vi "Main.vi"() -> ()   [LabVIEW 2018]
uses:
  Main_SubVI/Progress.vi
  <vilib>/Utility/file.llb/Write Delimited Spreadsheet (DBL).vi
panel:
  out "error out":errorcluster
  out "Progress Output":string
  out "Progress":u8(slide) scale=0.0..100.0
  out "Arduino Conn":bool
  in  "Arduino Connection":T1={"Baud rate (115200)"=115200, "VISA resource name"="", "Disconnect"=FALSE} {"Baud rate (115200)" min=38400 max=500000 step=1}
  out "Monitor":T2 {"Elapsed time [s]" format="%#_1g"}
  in  "Tab Plot":enum32{"Plot Measure", "Calibration Settings"}(tab)
  out "Measure VS Distance Reference":cluster{dbl[], dbl[]}(graph)
  out "Distance Sample":T3(graph)
  in  "Calibration":bool
  in  "Auto Validation":bool
  in  "Tare":bool
  in  "Reset Calibration":bool
  out "Calibration Curve":cluster{"Best Linear Fit":dbl[], dbl[]}[](graph)
  out "Calibration parameters":T4
  in  "Save Calibration":bool
  out "Measure":T5 {"Arduino distance [mm]" format="%#_5g"}
  in  "Tab Control":enum32{"Manual", " Programmable"}(tab)
  in  "Stop 2":bool
  out "Motor Ready":bool
  out "Communication\nAcknowledged":bool
  in  "Direction":bool
  in  "Motor relative position [mm]":dbl(knob) min=0.0 max=199.89999389648438 step=0.1 scale=0.0..100.0
  in  "Start Communication":bool
  in  "Samples per position":i32=1 min=1 step=1
  in  "Import":path
  in  "Start Auto Communication":bool
  in  "Stop":bool
  out "VISA resource name out":refnum<visa-resource-name>
  # "%"
  # "Up"
  # "Down"
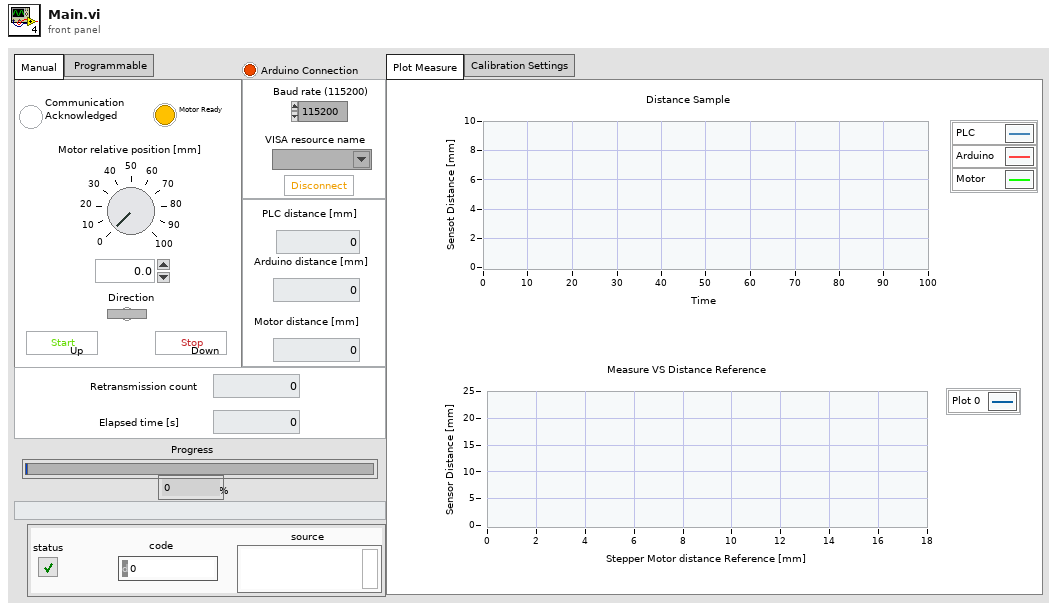
[diagram p1: front panel]
types:
  T1 = cluster{"Baud rate (115200)":u32, "VISA resource name":refnum<visa-resource-name>, "Disconnect":bool}
  T2 = cluster{"Elapsed time [s]":dbl, "Retransmission count":dbl}
  T3 = cluster{"PLC Sensor":dbl, "Arduino Sensor":dbl, "Position Reference":dbl}
  T4 = cluster{"Gain":dbl, "Offset":dbl, "ERMS":dbl, "STD":dbl, "Samples ":dbl}
  T5 = cluster{"PLC distance [mm] ":dbl, "Arduino distance [mm]":dbl, "Motor distance [mm]":dbl}
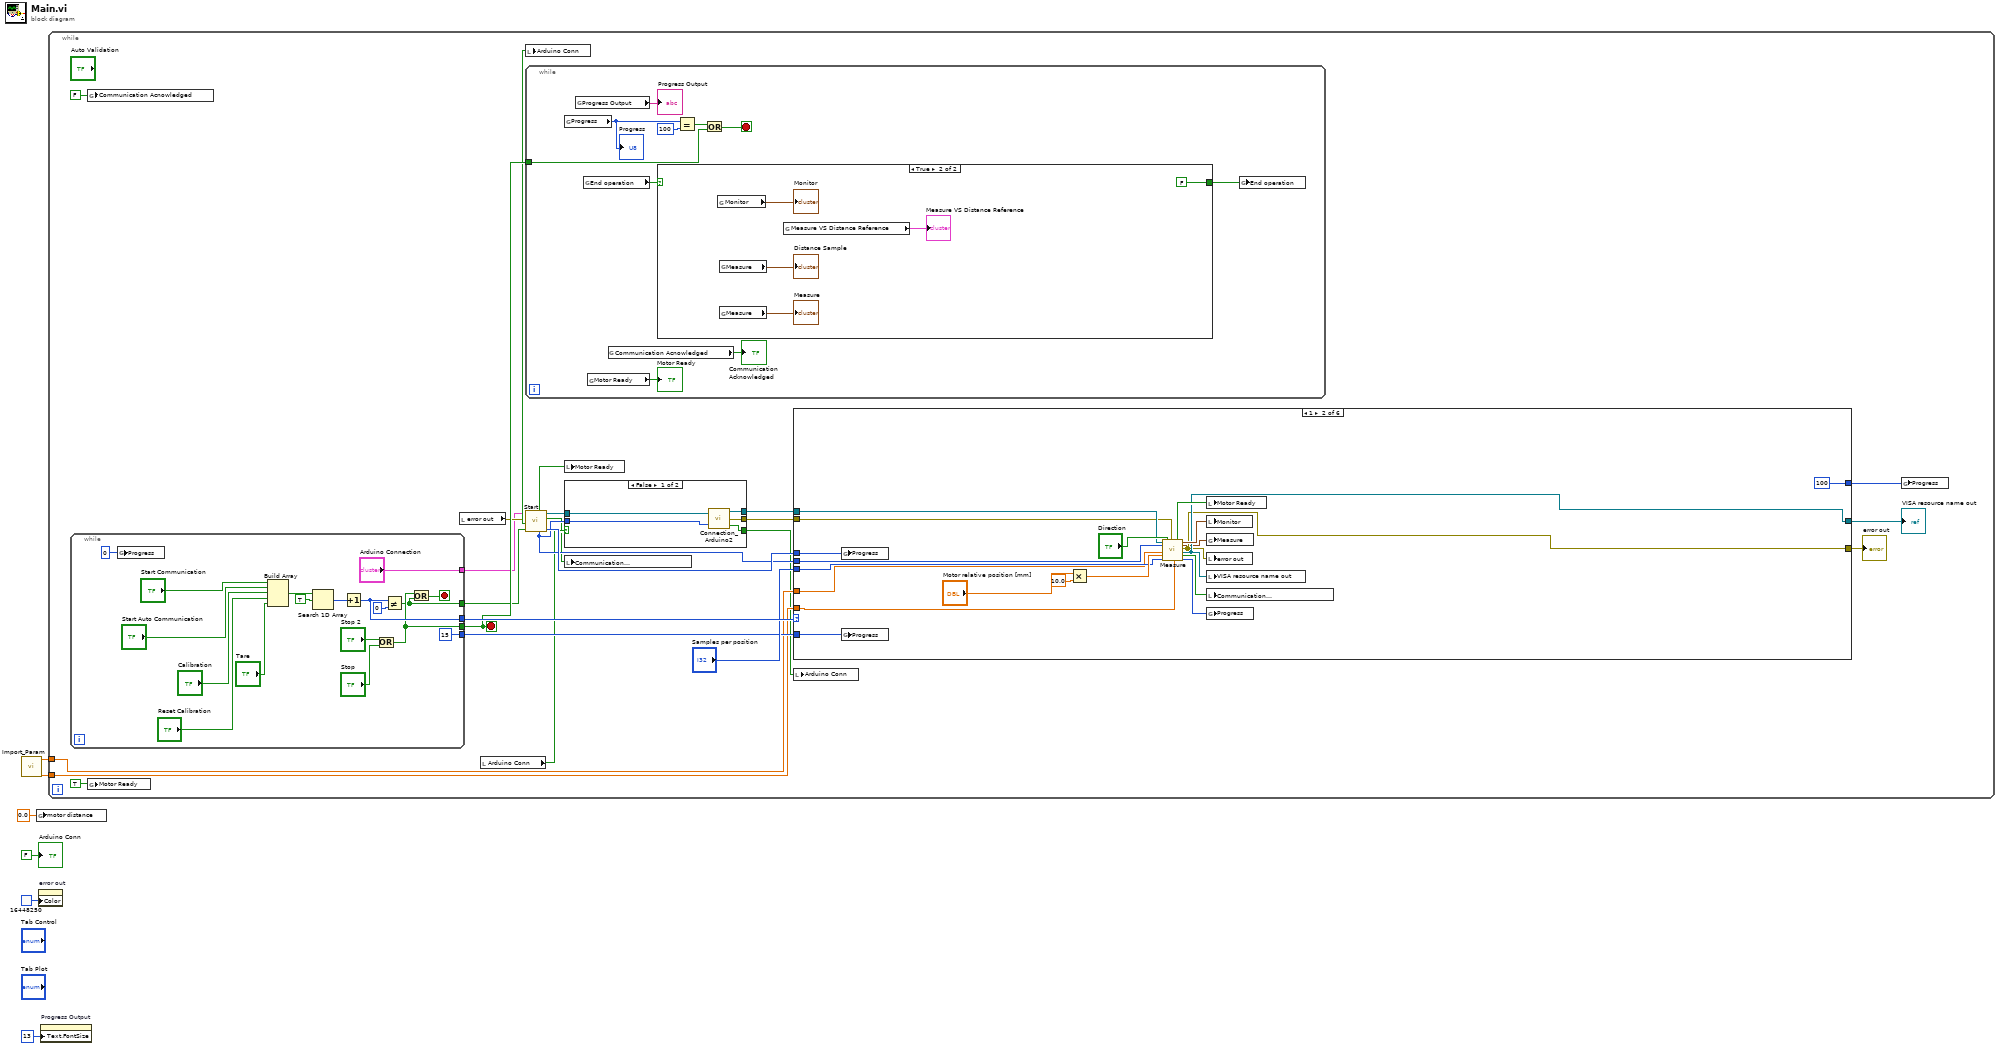
[diagram p0: block diagram]
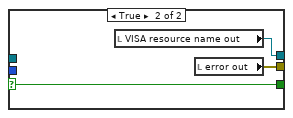
[diagram p2: hidden frame]
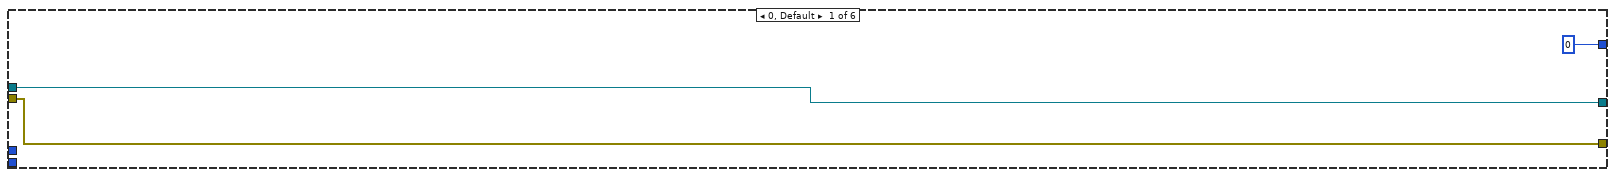
[diagram p3: hidden frame]
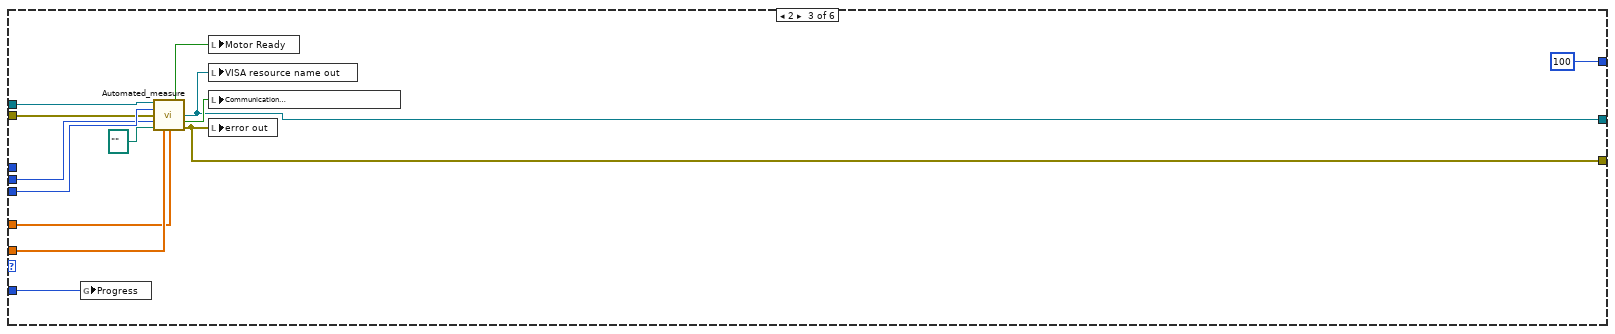
[diagram p4: hidden frame]
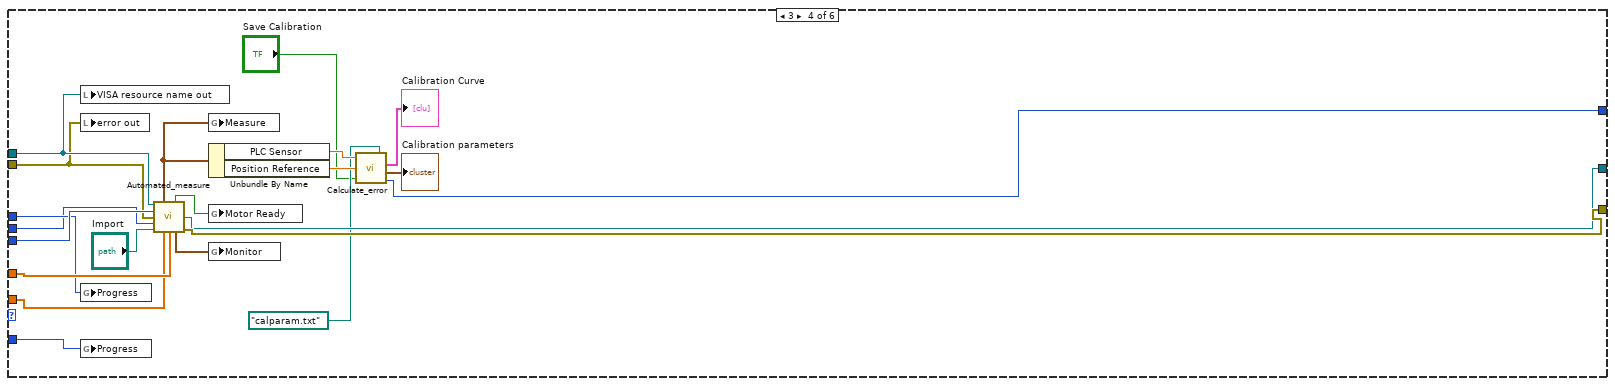
[diagram p5: hidden frame]
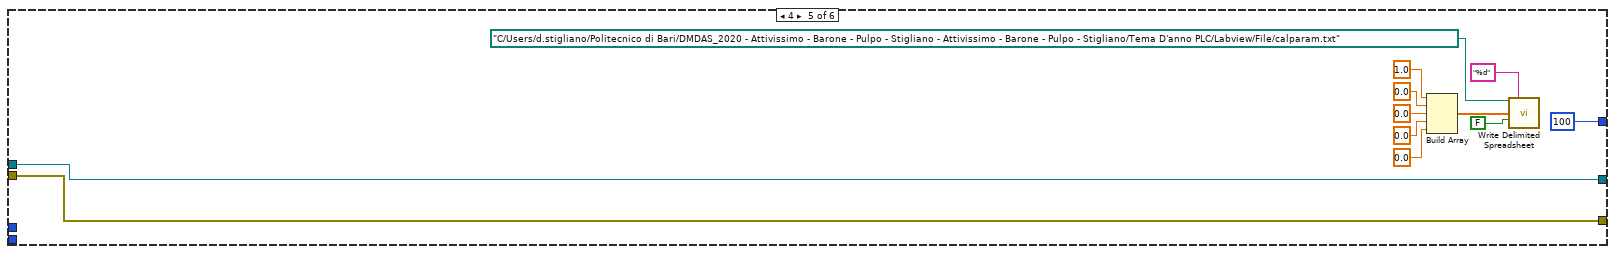
[diagram p6: hidden frame]
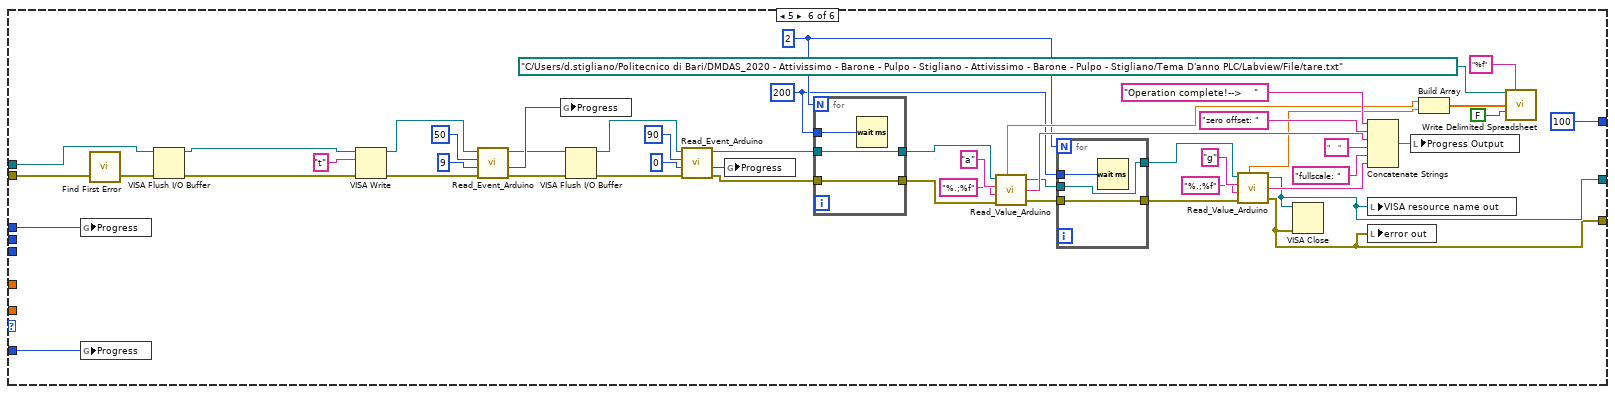
[diagram p7: hidden frame]
diagram:
  n1 = call "Import_Param.vi"() -> ("Calparam"=w5:sgl[], "Initial Tare"=w6:sgl[])  [unwired: 2 out]
  n2 = global write "Progress.vi" "motor distance"(0.0 ("motor distance")) -> ()
  n3 = property on="error out" class="Clust (strict)"("Color"=u32 16448250) -> ()  [unwired: 2 in, 2 out]
  n4 = property on="Progress Output" class="Str"("Text.FontSize"=u32 13 ("Text.Font:Size")) -> ()  [unwired: 2 in, 2 out]
  n5 = while {
    tunnel: w6 -> [w25]
    tunnel: w5 -> [w24]
    stop <- w28 stop-if-true
    n6 = while {
      tunnel: [u8 15 ("Slide")] -> w27
      tunnel: [w48] -> w30
      tunnel: [w43] -> w28
      tunnel: ["Arduino Connection"] -> w8
      tunnel: [w39] -> w7
      stop <- w40 stop-if-true
      n7 = global write "Progress.vi" "Progress"(u8 0 ("Slide")) -> ()
      n8 = Build Array("Start Communication", "Start Auto Communication", "Calibration", "Reset Calibration", "Tare") -> (w56:bool[])
      n9 = Search 1D Array(1D array=w56, element=TRUE) -> (index of element=w54:i32)  [unwired: 1 in]
      n10 = Increment(x=w54) -> (x+1=w48:i32)
      n11 = Or(x="Stop 2", y="Stop") -> (x .or. y?=w43:bool)
      n12 = Not Equal?(x=w48, y=0) -> (x != y?=w39:bool)
      n13 = Or(x=w43, y=w39) -> (x .or. y?=w40:bool)
    }
    n14 = global write "Progress.vi" "Communication Acnowledged"(FALSE ("Communication")) -> ()
    n15 = global write "Progress.vi" "Motor Ready"(TRUE ("Communication")) -> ()
    n16 = local read "error out"() -> (w9:errorcluster)
    n17 = local read "Arduino Conn"() -> (w15:bool)
    n18 = while {
      tunnel: w28 -> [w187]
      stop <- w189 stop-if-true
      n19 = global read "Progress.vi" "Progress"() -> (w191:u8)
      "Progress" <- w191
      n20 = global read "Progress.vi" "Progress Output"() -> (→"Progress Output":string)
      n21 = global read "Progress.vi" "End operation"() -> (w183:bool)
      n22 = global read "Progress.vi" "Motor Ready"() -> (→"Motor Ready":bool)
      n23 = global read "Progress.vi" "Communication Acnowledged"() -> (→"Communication\nAcknowledged":bool)
      n24 = case shown="True" w183 {
        selector: w183 -> [w192 _]
        tunnel: [w192 FALSE ("End operation")] -> w182
        frame False {
        }
        frame True {
          n25 = global read "Progress.vi" "Monitor"() -> (→"Monitor":T2)
          n26 = global read "Progress.vi" "Measure"() -> (→"Distance Sample":T5)
          n27 = global read "Progress.vi" "Measure"() -> (→"Measure":T5)
          n28 = global read "Progress.vi" "Measure VS Distance Reference"() -> (→"Measure VS Distance Reference":cluster{dbl[], dbl[]})
        }
      }
      n29 = Equal?(x=w191, y=u8 100) -> (x = y?=w188:bool)
      n30 = Or(x=w188, y=w187) -> (x .or. y?=w189:bool)
      n31 = global write "Progress.vi" "End operation"(w182) -> ()
    }
    n32 = call "Start.vi"("Arduino Connection"=w8, "error in (no error)"=w9, "Start Communication"=w7) -> ("Arduino Conn"=w17:bool, "Motor Ready"=w22:bool, "Baud rate (115200)"=w19:u32, "VISA resource name"=w16:refnum<visa-resource-name>, "Communication"=w14:bool, "Slide"=w23:u8)  [unwired: 1 out]
    n33 = local write "Arduino Conn"(w17) -> ()
    n34 = local write "Motor Ready"(w22) -> ()
    n35 = case shown="False" w15 {
      selector: w15 -> [_ w36]
      tunnel: w19 -> [w35 _]
      tunnel: [w34 w38] -> w20
      tunnel: [w33 w37] -> w21
      tunnel: [w32 w36] -> w18
      tunnel: w16 -> [w31 _]
      frame False {
        n36 = call "Connection_Arduino2.vi"("VISA resource name"=w31, "baud rate (9600)"=w35) -> ("VISA resource name out"=w34:refnum<visa-resource-name>, "error out"=w33:errorcluster, "Arduino Conn"=w32:bool)
      }
      frame True {
        n37 = local read "VISA resource name out"() -> (w38:refnum<visa-resource-name>)
        n38 = local read "error out"() -> (w37:errorcluster)
      }
    }
    n39 = local write "Communication\nAcknowledged"(w14) -> ()
    n40 = case shown="1" w30 {
      tunnel: "Samples per position" -> [_ w74 w90 w112 _ _]
      tunnel: w27 -> [_ w73 w89 w111 _ w169]
      tunnel: [u8 0 ("Progress") u8 100 ("Progress") u8 100 ("Progress") w93 u8 100 ("Progress") u8 100 ("Progress")] -> w26
      tunnel: w25 -> [_ w72 w86 w110 _ _]
      tunnel: w24 -> [_ w71 w87 w109 _ _]
      tunnel: w23 -> [_ w70 _ w108 _ w130]
      tunnel: w20 -> [w58 w69 w81 w106 w115 w129]
      tunnel: w21 -> [w57 w67 w83 w105 w114 w128]
      tunnel: w19 -> [_ w68 w84 w107 _ _]
      tunnel: [w57 w63 w82 w103 w114 w126] -> w13
      tunnel: [w58 w64 w80 w102 w115 w127] -> w12
      frame 0, Default {
      }
      frame 1 {
        n41 = global write "Progress.vi" "Progress"(w70) -> ()
        n42 = global write "Progress.vi" "Progress"(w73) -> ()
        n43 = Multiply(x="Motor relative position [mm]", y=10.0) -> (x*y=w79:dbl)
        n44 = call "Measure.vi"("VISA resource name"=w69, "Baud rate (115200)"=w68, "Initial Tare"=w72, "Motor relative position"=w79, "Samples per position"=w74, "Direction"="Direction", "error in"=w67, "Cal Param"=w71) -> ("Motor Ready"=w66:bool, "Monitor"=w77:T2, "Measure"=w62:T5, "error out"=w63:errorcluster, "VISA resource name out"=w64:refnum<visa-resource-name>, "Communication\nAcknowledged"=w65:bool, "Progress"=w61:u8)  [unwired: 5 in]
        n45 = local write "Motor Ready"(w66) -> ()
        n46 = local write "Monitor"(w77) -> ()
        n47 = global write "Progress.vi" "Measure"(w62) -> ()
        n48 = local write "error out"(w63) -> ()
        n49 = local write "VISA resource name out"(w64) -> ()
        n50 = local write "Communication\nAcknowledged"(w65) -> ()
        n51 = global write "Progress.vi" "Progress"(w61) -> ()
      }
      frame 2 {
        n52 = global write "Progress.vi" "Progress"(w89) -> ()
        n53 = call "Automated_measure.vi"("VISA resource name"=w81, "Samples per position"=w90, "error in"=w83, "Baud rate (115200)"=w84, "Import"=path "", "Cal Param"=w87, "Initial Tare"=w86) -> ("Motor Ready"=w92:bool, "VISA resource name out"=w80:refnum<visa-resource-name>, "Communication OK"=w85:bool, "error out"=w82:errorcluster)  [unwired: 3 in, 2 out]
        n54 = local write "Motor Ready"(w92) -> ()
        n55 = local write "VISA resource name out"(w80) -> ()
        n56 = local write "Communication\nAcknowledged"(w85) -> ()
        n57 = local write "error out"(w82) -> ()
      }
      frame 3 {
        n58 = local write "VISA resource name out"(w106) -> ()
        n59 = local write "error out"(w105) -> ()
        n60 = global write "Progress.vi" "Progress"(w108) -> ()
        n61 = global write "Progress.vi" "Progress"(w111) -> ()
        n62 = call "Automated_measure.vi"("VISA resource name"=w106, "Samples per position"=w112, "error in"=w105, "Baud rate (115200)"=w107, "Import"="Import", "Cal Param"=w109, "Initial Tare"=w110) -> ("Measure"=w94:T3, "Motor Ready"=w104:bool, "VISA resource name out"=w102:refnum<visa-resource-name>, "Monitor"=w101:T2, "error out"=w103:errorcluster)  [unwired: 3 in, 1 out]
        n63 = global write "Progress.vi" "Measure"(w94) -> ()
        n64 = Unbundle By Name(w94) -> ("PLC Sensor"=w97:dbl, "Position Reference"=w98:dbl)
        n65 = global write "Progress.vi" "Motor Ready"(w104) -> ()
        n66 = global write "Progress.vi" "Monitor"(w101) -> ()
        n67 = call "Calculate_error.vi"("x 2"=w97, "x 1"=w98, "Button"="Save Calibration", "file path (dialog if empty)"=path "calparam.txt") -> ("Calibration Curve"=→"Calibration Curve":cluster{"Best Linear Fit":dbl[], dbl[]}[], "Calibration parameters"=→"Calibration parameters":T4, "Slide"=w93:u8)
      }
      frame 4 {
        n68 = Build Array(1.0 ("element"), 0.0 ("element"), 0.0 ("element"), 0.0 ("element"), 0.0 ("element")) -> (w116:dbl[])
        n69 = call-poly <vilib>:"Write Delimited Spreadsheet.vi"("file path (dialog if empty)"=path "C:/Users/d.stigliano/Politecnico di Bari/DMDAS_2020 - Attivissimo - Barone - Pulpo - Stigliano - Attivissimo - Barone - Pulpo - Stigliano/Tema D'anno PLC/Labview/File/calparam.txt", "format (%.3f)"="%d", "1D data"=w116, "append to file? (new file:F)"=FALSE) -> ()  [unwired: 10 in, 2 out]
      }
      frame 5 {
        w133 = u32 200 ("milliseconds to wait")
        w135 = 2
        n70 = global write "Progress.vi" "Progress"(w130) -> ()
        n71 = global write "Progress.vi" "Progress"(w169) -> ()
        n72 = call <vilib>:"Find First Error.vi"("error in (no error)"=w128) -> ("error out"=w172:errorcluster)  [unwired: 3 in, 1 out]
        n73 = VISA Flush I/O Buffer(VISA resource name=w129, error in (no error)=w172) -> (VISA resource name out=w168:refnum<visa-resource-name>, error out=w171:errorcluster)  [unwired: 1 in]
        n74 = VISA Write(VISA resource name=w168, write buffer="t", error in (no error)=w171) -> (VISA resource name out=w165:refnum<visa-resource-name>, error out=w164:errorcluster)  [unwired: 1 out]
        n75 = call "Read_Event_Arduino.vi"("error in"=w164, "condition"=9, "Progress in"=u8 50 ("Progress"), "VISA resource name in"=w165) -> ("error out"=w155:errorcluster, "Progress"=w163:u8, "VISA resource name out"=w157:refnum<visa-resource-name>)  [unwired: 4 in, 1 out]
        n76 = global write "Progress.vi" "Progress"(w163) -> ()
        n77 = VISA Flush I/O Buffer(VISA resource name=w157, error in (no error)=w155) -> (VISA resource name out=w156:refnum<visa-resource-name>, error out=w154:errorcluster)  [unwired: 1 in]
        n78 = call "Read_Event_Arduino.vi"("error in"=w154, "condition"=0, "Progress in"=u8 90, "VISA resource name in"=w156) -> ("error out"=w143:errorcluster, "Progress"=w162:u8, "VISA resource name out"=w146:refnum<visa-resource-name>)  [unwired: 4 in, 1 out]
        n79 = global write "Progress.vi" "Progress"(w162) -> ()
        n80 = for {
          N: w135 -> [_]
          tunnel: w146 -> [w181]
          tunnel: [w181] -> w145
          tunnel: [w180] -> w144
          tunnel: w143 -> [w180]
          tunnel: w133 -> [w179]
          n81 = Wait (ms)(milliseconds to wait=w179) -> ()  [unwired: 1 out]
        }
        n82 = call "Read_Value_Arduino.vi"("VISA resource name"=w145, "write buffer"="a", "format string (%.;%f)"="%.;%f" ("format string (%d)"), "error in (no error)"=w144) -> ("output"=w147:dbl, "VISA resource name out"=w142:refnum<visa-resource-name>, "concatenated string"=w149:string, "error out"=w141:errorcluster)
        n83 = for {
          N: w135 -> [_]
          tunnel: w142 -> [w177]
          tunnel: [w178] -> w140
          tunnel: w141 -> [w178]
          tunnel: [w177] -> w139
          tunnel: w133 -> [w176]
          n84 = Wait (ms)(milliseconds to wait=w176) -> ()  [unwired: 1 out]
        }
        n85 = call "Read_Value_Arduino.vi"("VISA resource name"=w139, "write buffer"="g", "format string (%.;%f)"="%.;%f" ("format string (%d)"), "error in (no error)"=w140) -> ("output"=w148:dbl, "VISA resource name out"=w127:refnum<visa-resource-name>, "concatenated string"=w138:string, "error out"=w126:errorcluster)
        n86 = VISA Close(VISA resource name=w127, error in (no error)=w126) -> ()  [unwired: 1 out]
        n87 = Concatenate Strings("Operation complete!-->    " ("string"), "zero offset: " ("string"), w149, "    " ("string"), "fullscale: " ("string"), w138) -> (w132:string)
        n88 = local write "VISA resource name out"(w127) -> ()
        n89 = local write "error out"(w126) -> ()
        n90 = local write "Progress Output"(w132) -> ()
        n91 = Build Array(w147, w148) -> (w131:dbl[])
        n92 = call-poly <vilib>:"Write Delimited Spreadsheet.vi"("file path (dialog if empty)"=path "C:/Users/d.stigliano/Politecnico di Bari/DMDAS_2020 - Attivissimo - Barone - Pulpo - Stigliano - Attivissimo - Barone - Pulpo - Stigliano/Tema D'anno PLC/Labview/File/tare.txt", "format (%.3f)"="%f", "1D data"=w131, "append to file? (new file:F)"=FALSE) -> ()  [unwired: 10 in, 2 out]
      }
    }
    "error out" <- w13
    "VISA resource name out" <- w12
    n93 = local write "Arduino Conn"(w18) -> ()
    n94 = global write "Progress.vi" "Progress"(w26) -> ()
  }
  "Arduino Conn" <- FALSE ("Arduino Conn")
